vi "Do.vi"(8 "error in (no error)":errorcluster, 10 "Actor in":refnum<class "Actor.lvclass">, 11 "Open menu object parameters Msg":refnum<class "Open menu object parameters Msg.lvclass">) -> (0 "error out":errorcluster, 2 "Actor out":refnum<class "Actor.lvclass">)   [LabVIEW 2015, in "Open menu object parameters Msg.lvclass"]
doc: "This VI delivers the message to the actor by calling the appropriate method(s) on the actor."
uses:
  Open menu object parameters Msg.lvclass
  <vilib>/ActorFramework/Actor/Actor.lvclass
  Mag Lab Measure Interface/Mag Lab Measure UI.lvclass
  Open menu object parameters Msg.lvclass/Open menu object parameters Msg.ctl
  Mag Lab Error Handler/Mag Lab Error Handler.lvclass
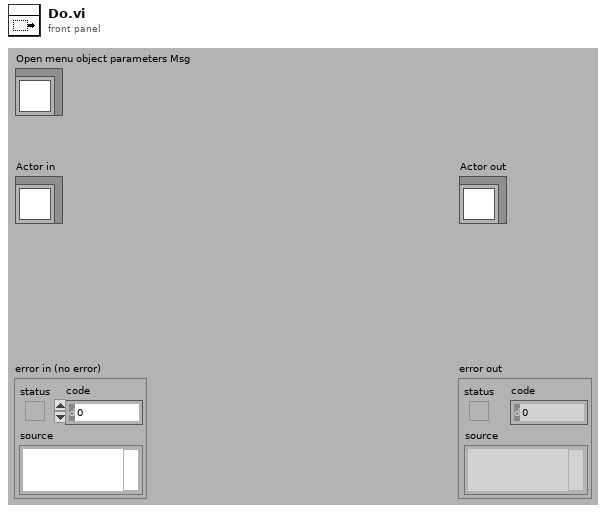
[diagram p1: front panel]
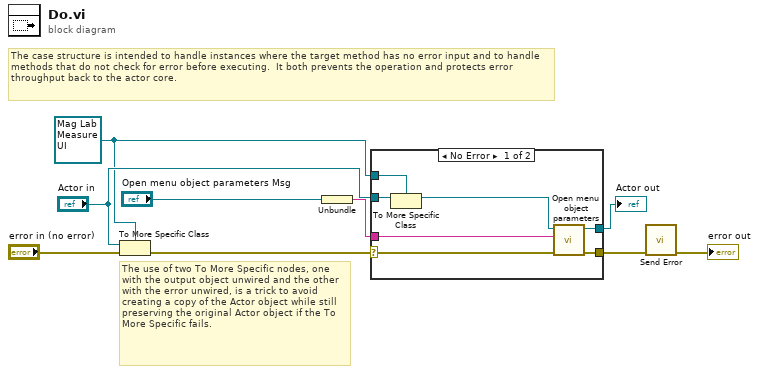
[diagram p0: block diagram]
diagram:
  w4 = refnum<class "Mag Lab Measure UI.lvclass"> refnum ("Actor in")
  # "The use of two To More Specific nodes, one with the output object unwired and the other with the error unwired, is a trick to avoid creating a copy of the Actor object while still preserving the original Actor object if the To More Specific fails."
  # "The case structure is intended to handle instances where the target method has no error input and to handle methods that do not check for error before executing.  It both prevents the operation and protects error throughput back to the actor core."
  n1 = To More Specific Class(target class=w4, reference="Actor in", error in="error in (no error)") -> (error out=w7:errorcluster)  [unwired: 1 out]
  n2 = Unbundle("Open menu object parameters Msg") -> (w3:string)
  n3 = case shown="No Error" w7 {
    selector: w7 -> [w14 w18]
    tunnel: [w16 w18] -> w2
    tunnel: [w15 w17] -> w6
    tunnel: "Actor in" -> [w13 w17]
    tunnel: w4 -> [w12 _]
    tunnel: w3 -> [w10 _]
    frame No Error {
      n4 = To More Specific Class(target class=w12, reference=w13) -> (specific class reference=w11:refnum<class "Mag Lab Measure UI.lvclass">)  [unwired: 1 in, 1 out]
      n5 = call-dynamic "Open menu object parameters.vi"("error in (no error)"=w14, "Object name"=w10, "Mag Lab Measure Interface in"=w11) -> ("error out"=w16:errorcluster, "Mag Lab Measure Interface out"=w15:refnum<class "Mag Lab Measure UI.lvclass">)  [unwired: 7 in]
    }
    frame Error {
      # "If type check fails, pass the original object out again."
    }
  }
  "Actor out" <- w6
  n6 = call "Send Error.vi"("error in (no error)"=w2) -> ("error out"=→"error out":errorcluster)  [unwired: 9 in, 1 out]
